vi "Hitronics.Main.vi"() -> ()   [LabVIEW 2020]
uses:
  VarsIn.ctl
  VarsOut.ctl
  State.ctl
  Agilent 2000 3000 X-Series/Agilent 2000 3000 X-Series.lvlib
panel:
  out "VarsOut":T1 {"Pk-Pk" format="%_6f"; "Delay 1-2" format="%_6f"; "Rise" format="%_6f"; "Width" format="%_6f"; "Power Value#2" format="%_6f"; "Power Value#1" format="%_6f"}
  out "error out":errorcluster
  in  "error in (no error)":errorcluster
  in  "VarsIn":T2 {"Pk-Pk" format="%_6f"; "Delay 1-2" format="%_6f"; "Rise" format="%_6f"; "Width" format="%_6f"; "Power Value#2" format="%_6f"; "Power Value#1" format="%_6f"}
  in  "Stop":bool
  in  "Test":bool=TRUE
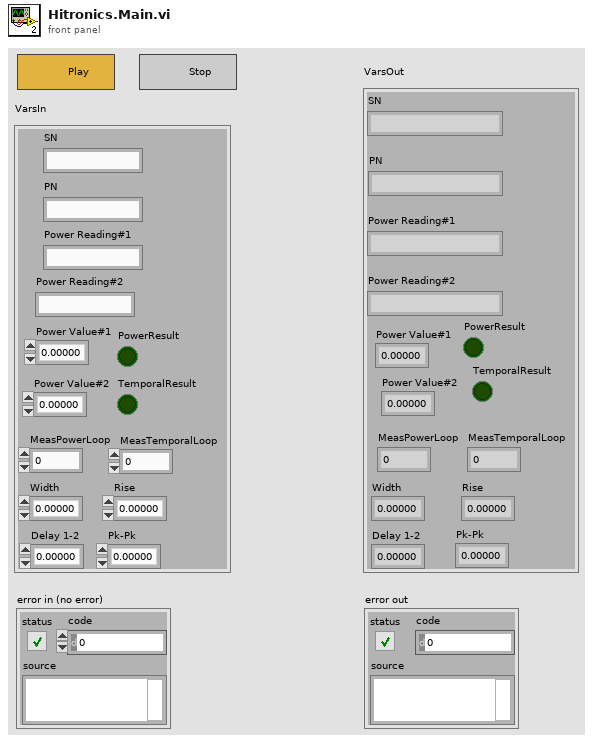
[diagram p1: front panel]
types:
  T1 = typedef "VarsOut.ctl" = cluster{"Power Reading#1":string, "Power Reading#2":string, "SN":string, "PN":string, "Power Value#1":dbl, "Power Value#2":dbl, "MeasPowerLoop":i16, "PowerResult":bool, "Width":dbl, "Rise":dbl, "Delay 1-2":dbl, "Pk-Pk":dbl, "TemporalResult":bool, "MeasTemporalLoop":i16}
  T2 = typedef "VarsIn.ctl" = cluster{"Power Reading#1":string, "Power Reading#2":string, "SN":string, "PN":string, "Power Value#1":dbl, "Power Value#2":dbl, "MeasPowerLoop":i16, "PowerResult":bool, "Width":dbl, "Rise":dbl, "Delay 1-2":dbl, "Pk-Pk":dbl, "TemporalResult":bool, "MeasTemporalLoop":i16}
  T3 = typedef "State.ctl" = enum16{"Init GUI", "ScanLabel", "MeasPower", "CheckPower", "MeasTemporal", "CheckTemporal", "Results", "SaveTestLog", "Close", "Open", "Process"}
  T4 = enum32{"invalid app kind", "Development System", "Run Time System", "Student Edition", "Embedded LabVIEW", "Evaluation", "Custom"}
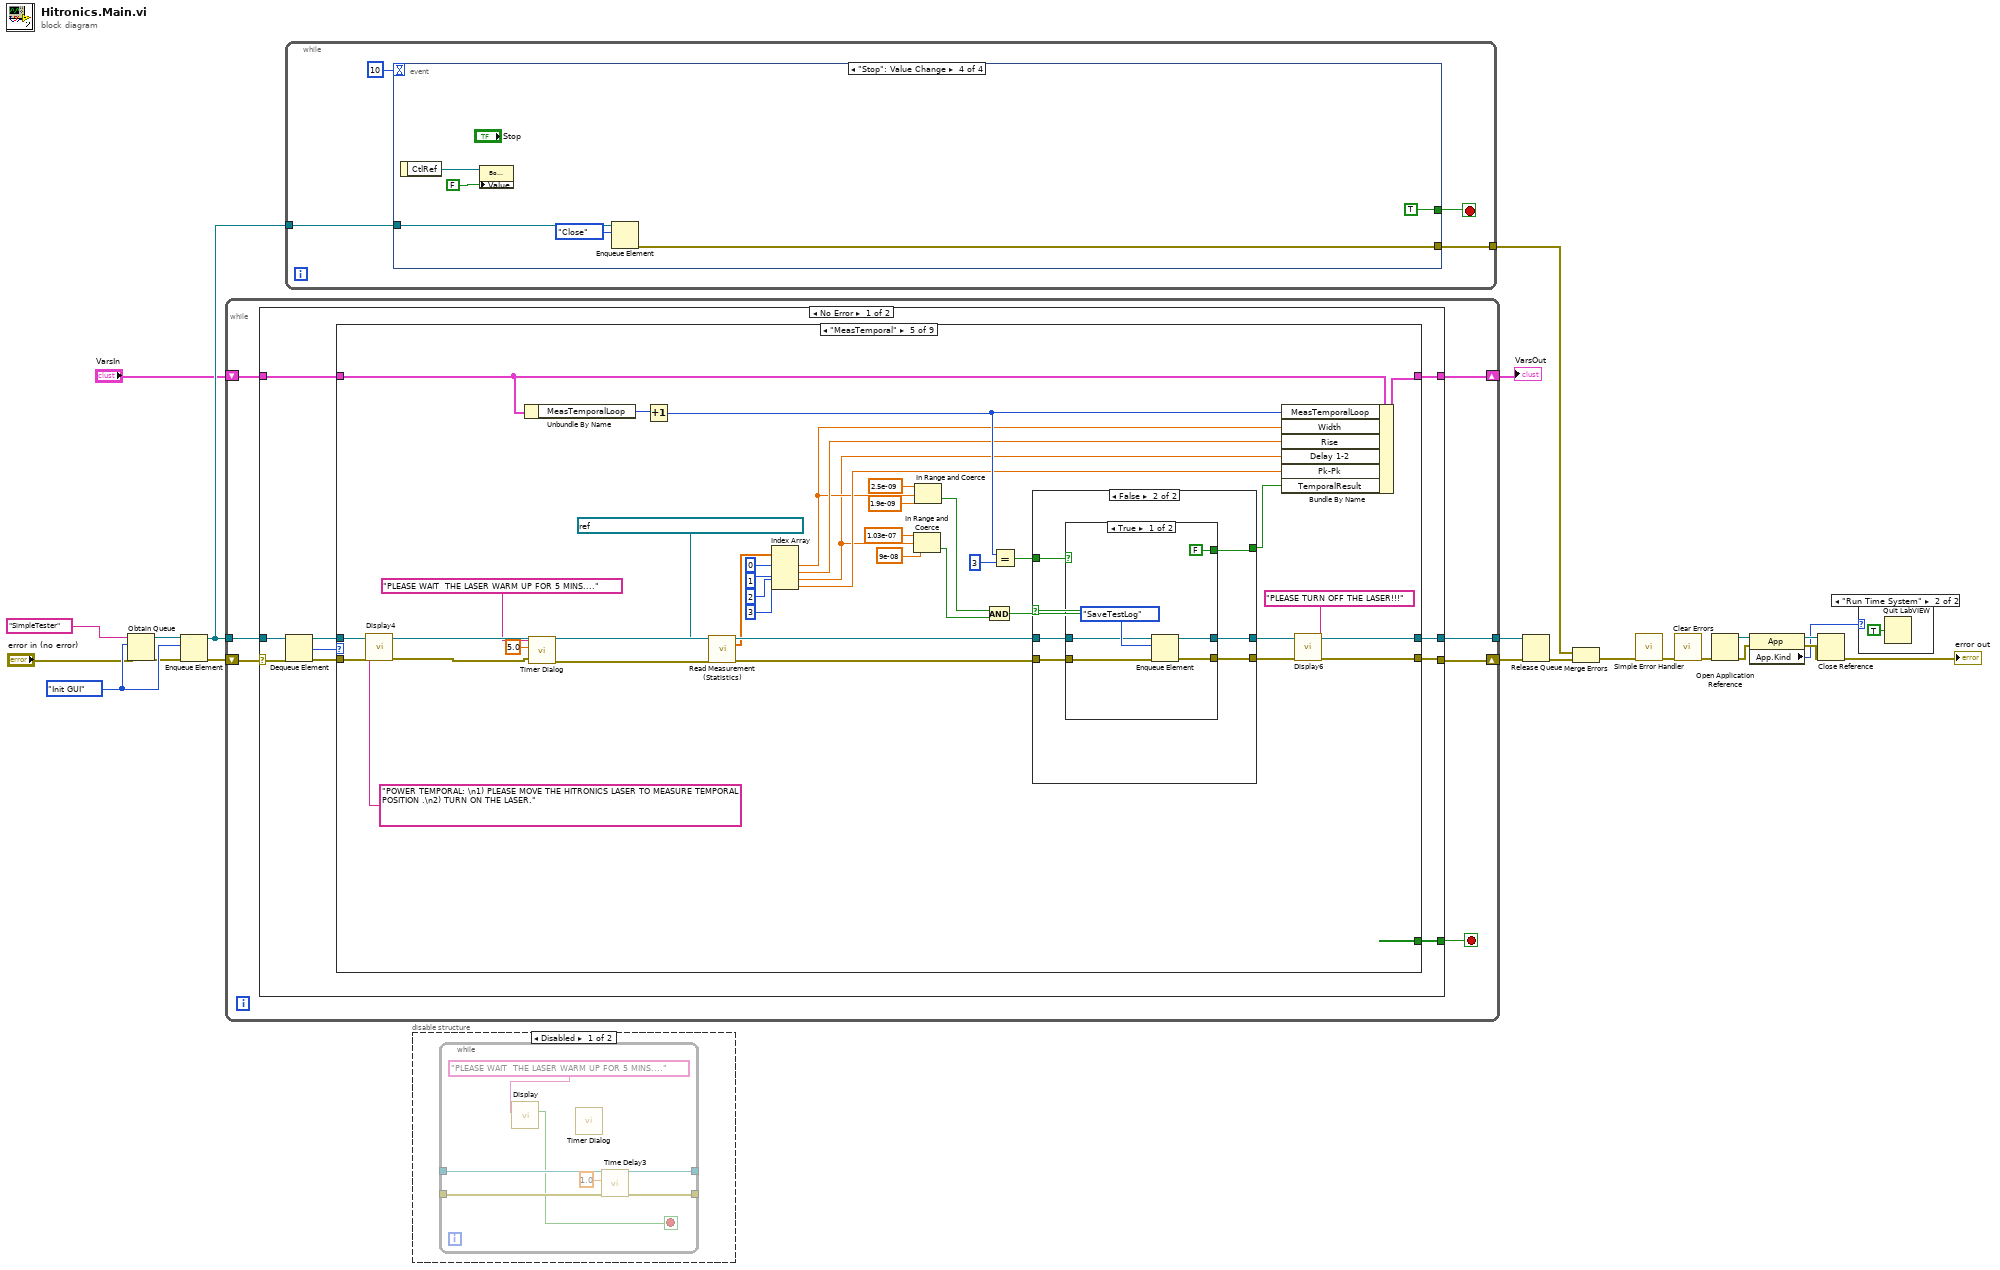
[diagram p0: block diagram]
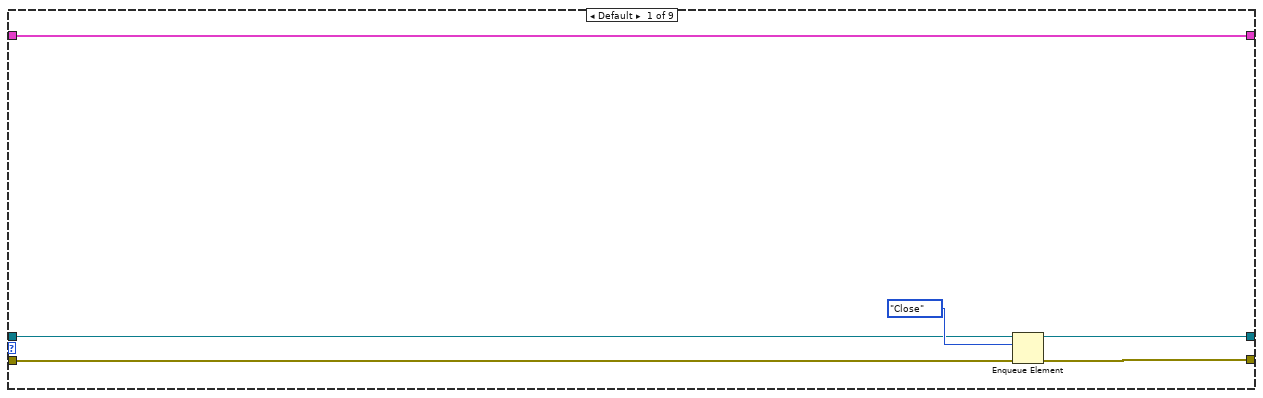
[diagram p4: hidden frame]
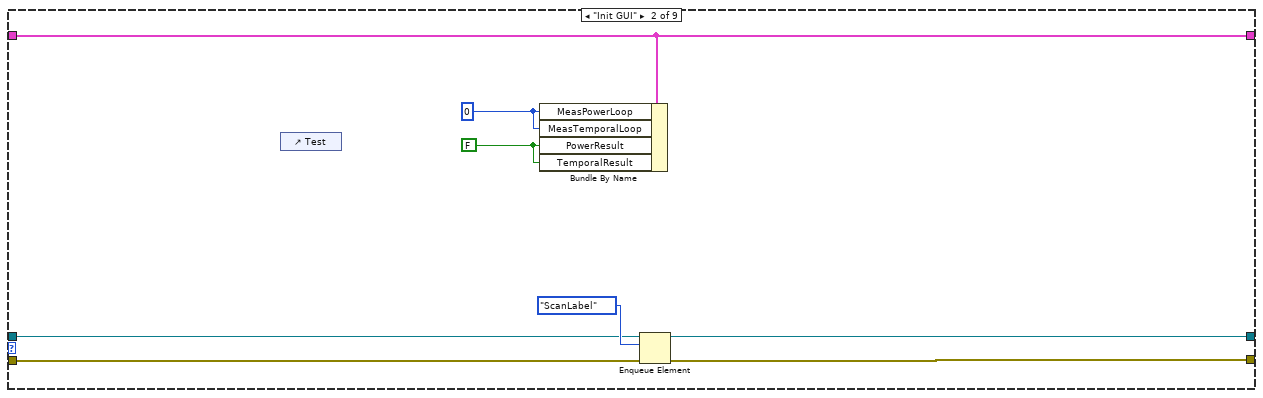
[diagram p5: hidden frame]
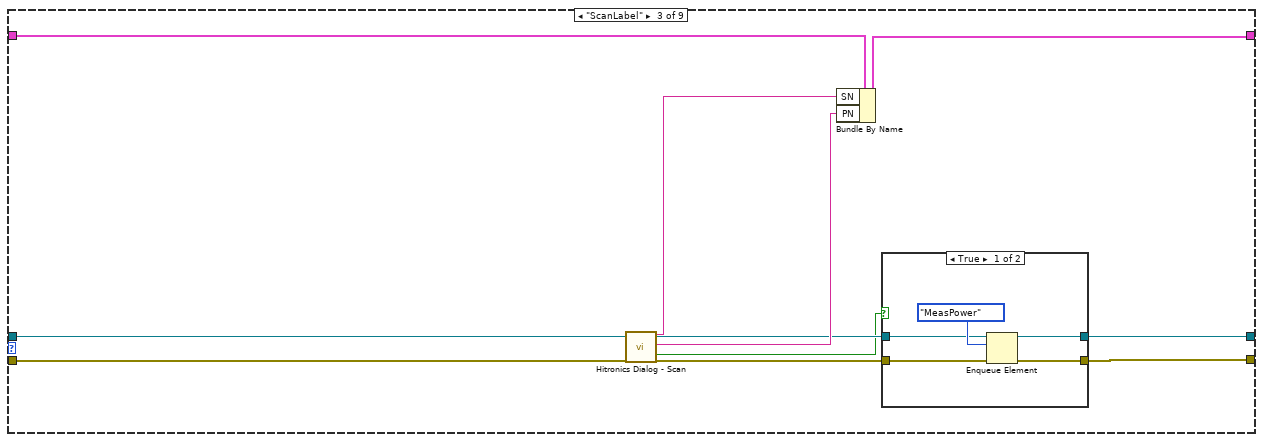
[diagram p6: hidden frame]
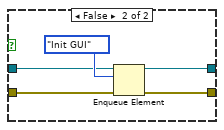
[diagram p7: hidden frame]
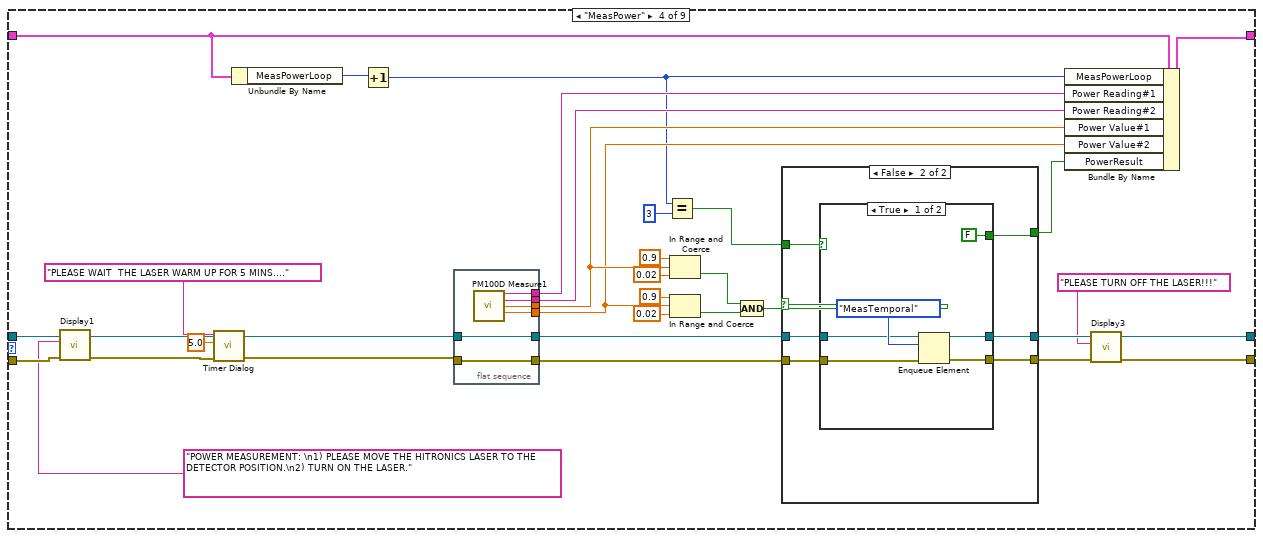
[diagram p8: hidden frame]
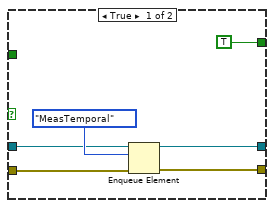
[diagram p9: hidden frame]
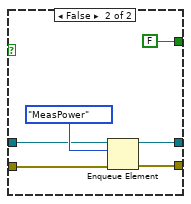
[diagram p10: hidden frame]
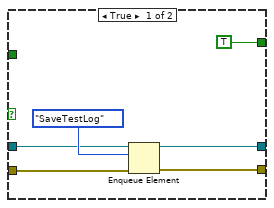
[diagram p11: hidden frame]
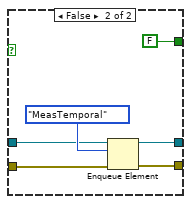
[diagram p12: hidden frame]
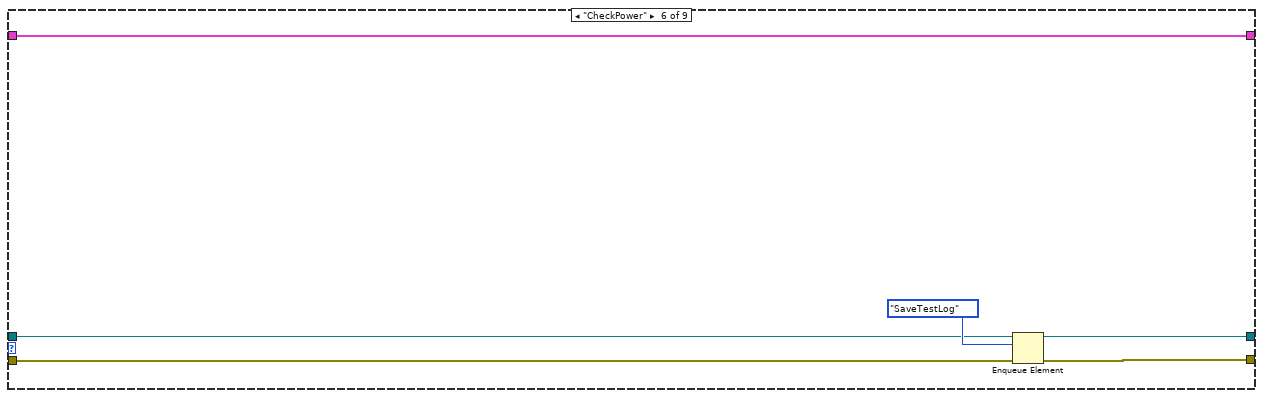
[diagram p13: hidden frame]
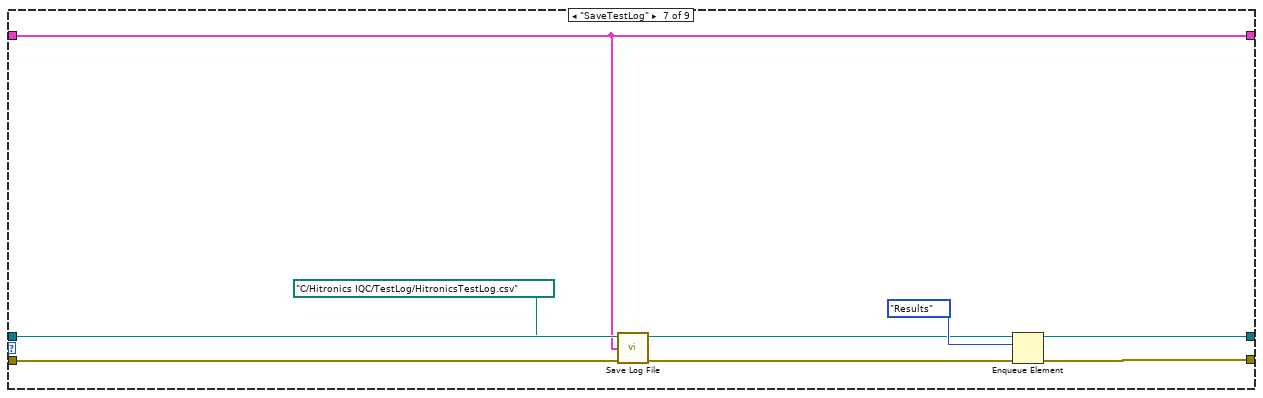
[diagram p14: hidden frame]
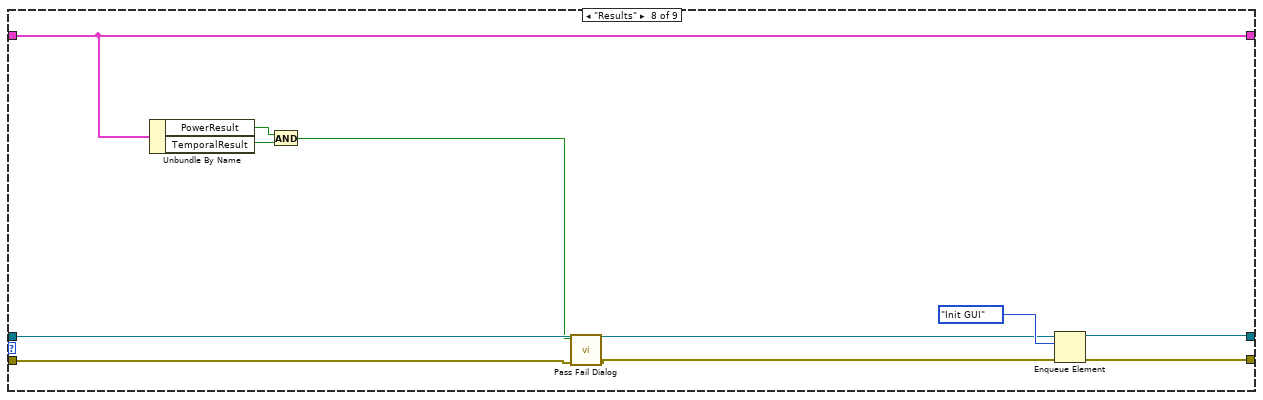
[diagram p15: hidden frame]
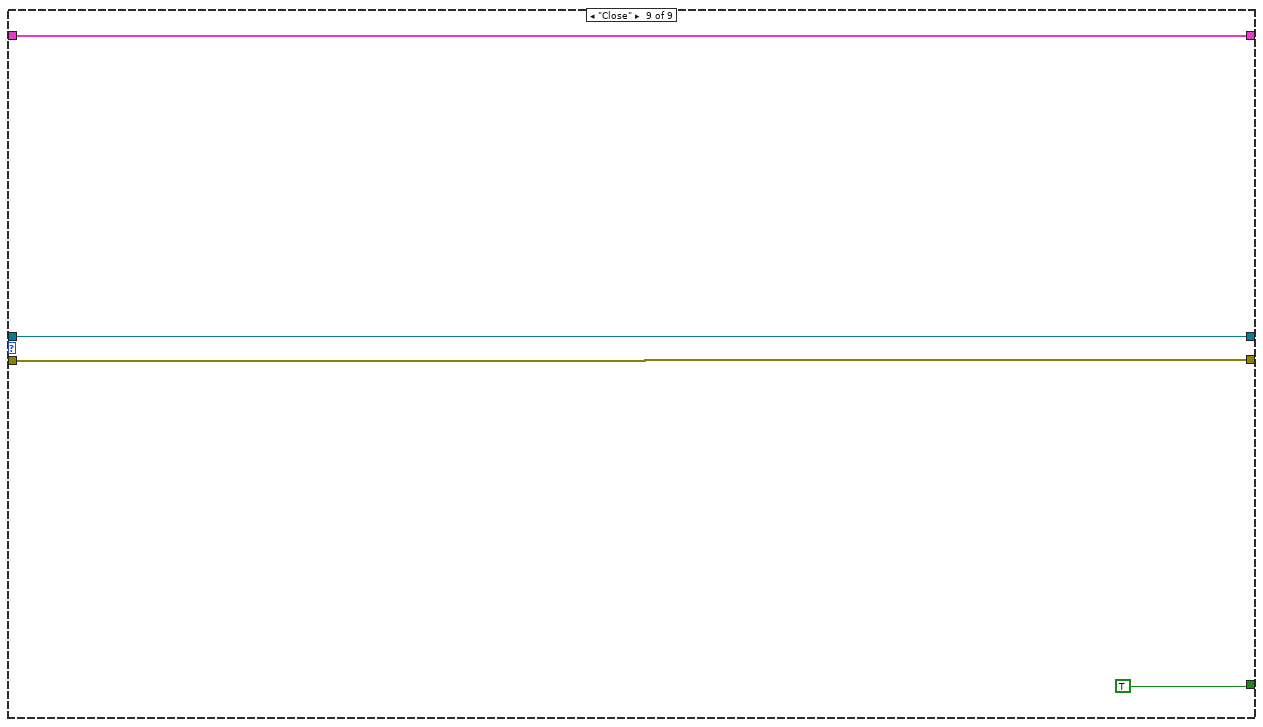
[diagram p16: hidden frame]
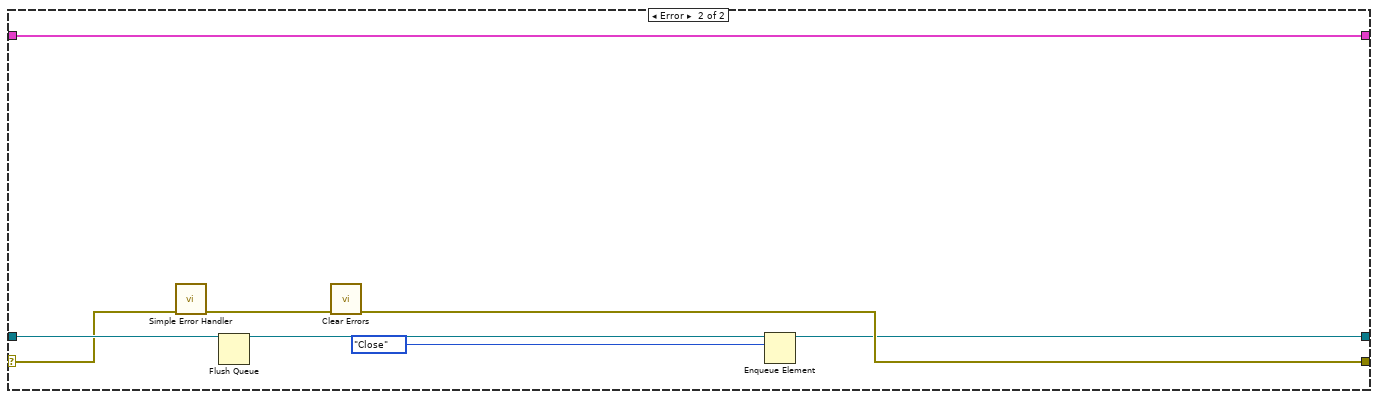
[diagram p17: hidden frame]
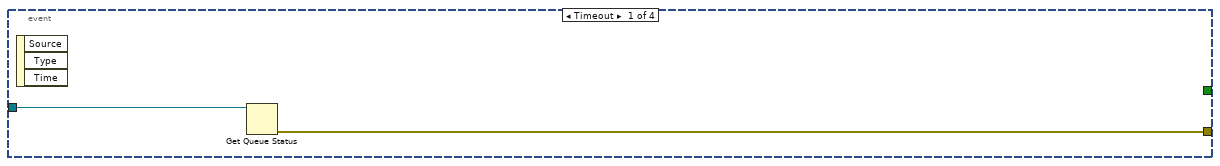
[diagram p18: hidden frame]
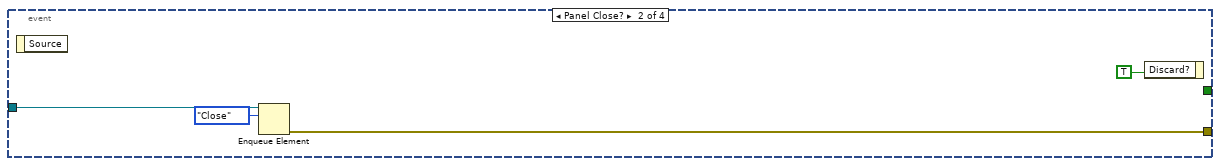
[diagram p19: hidden frame]
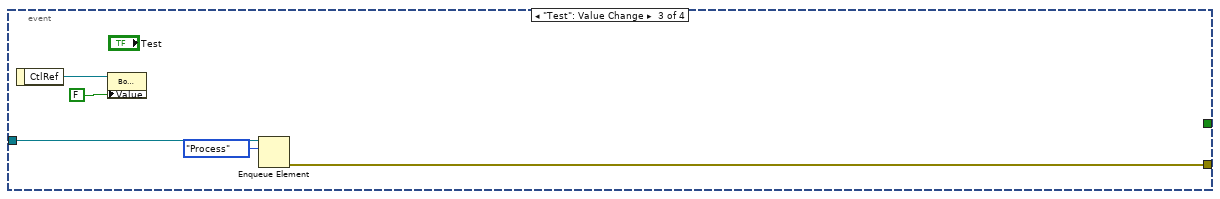
[diagram p20: hidden frame]
diagram:
  w12 = State."Init GUI"
  n1 = Obtain Queue(name (unnamed)="SimpleTester", element data type=w12, error in (no error)="error in (no error)") -> (queue out=w21:refnum<queue>, error out=w3:errorcluster)  [unwired: 2 in, 1 out]
  n2 = Enqueue Element(queue=w21, element=w12, error in (no error)=w3) -> (queue out=w19:refnum<queue>, error out=w4:errorcluster)  [unwired: 1 in, 1 out]
  n3 = while {
    tunnel: [w28] -> w20
    tunnel: w19 -> [w29]
    shift-right: [w25] -> w5
    shift-left: w4 -> [w26]
    shift-right: [w23] -> w1
    shift-left: "VarsIn" -> [w24]
    stop <- w27 stop-if-true
    n4 = case shown="No Error" w26 {
      selector: w26 -> [w32 w229]
      tunnel: w29 -> [w39 w230]
      tunnel: [w38 w224] -> w28
      tunnel: [w35 _] -> w27
      tunnel: [w30 w227] -> w25
      tunnel: [w34 w223] -> w23
      tunnel: w24 -> [w33 w223]
      frame No Error {
        n5 = Dequeue Element(queue=w39, error in (no error)=w32) -> (queue out=w37:refnum<queue>, element=w36:T3, error out=w31:errorcluster)  [unwired: 1 in, 1 out]
        n6 = case shown="\"MeasTemporal\"" w36 {
          tunnel: [w40 w49 w55 w104 w170 w197 w205 w216 w222] -> w38
          tunnel: w37 -> [w41 w50 w56 w76 w169 w198 w206 w212 w222]
          tunnel: [_ _ _ _ _ _ _ _ TRUE] -> w35
          tunnel: [w45 w48 w61 w101 w168 w196 w202 w215 w220] -> w34
          tunnel: w33 -> [w45 w48 w62 w87 w165 w196 w202 w215 w220]
          tunnel: w31 -> [w43 w52 w63 w98 w139 w195 w204 w214 w219]
          tunnel: [w42 w51 w57 w80 w140 w199 w207 w218 w219] -> w30
          frame Default {
            n7 = Enqueue Element(queue=w41, element=State."Close", error in (no error)=w43) -> (queue out=w40:refnum<queue>, error out=w42:errorcluster)  [unwired: 1 in, 1 out]
          }
          frame "Init GUI" {
            w46 = FALSE ("PowerResult")
            w47 = 0 ("MeasPowerLoop")
            n8 = control-ref of="Test"() -> ()  [unwired: 1 out]
            n9 = Bundle By Name(cluster=w48, "MeasPowerLoop"=w47, "MeasTemporalLoop"=w47, "PowerResult"=w46, "TemporalResult"=w46) -> ()  [unwired: 1 out]
            n10 = Enqueue Element(queue=w50, element=State."ScanLabel", error in (no error)=w52) -> (queue out=w49:refnum<queue>, error out=w51:errorcluster)  [unwired: 1 in, 1 out]
          }
          frame "ScanLabel" {
            n11 = call "Hitronics Dialog - Scan.vi"("error in (no error)"=w63) -> ("Serial Number"=w60:string, "Part Number"=w59:string, "Continue Exec?"=w54:bool, "error out"=w58:errorcluster)  [unwired: 14 in, 1 out]
            n12 = Bundle By Name(cluster=w62, "SN"=w60, "PN"=w59) -> (w61:T2)
            n13 = case shown="True" w54 {
              tunnel: w58 -> [w67 w72]
              tunnel: [w66 w71] -> w57
              tunnel: w56 -> [w65 w70]
              tunnel: [w64 w69] -> w55
              frame True {
                n14 = Enqueue Element(queue=w65, element=State."MeasPower", error in (no error)=w67) -> (queue out=w64:refnum<queue>, error out=w66:errorcluster)  [unwired: 1 in, 1 out]
              }
              frame False {
                n15 = Enqueue Element(queue=w70, element=State."Init GUI", error in (no error)=w72) -> (queue out=w69:refnum<queue>, error out=w71:errorcluster)  [unwired: 1 in, 1 out]
              }
            }
          }
          frame "MeasPower" {
            n16 = call "Display1"("error in (no error)"=w98, "Message"="POWER MEASUREMENT: \n1) PLEASE MOVE THE HITRONICS LASER TO THE DETECTOR POSITION.\n2) TURN ON THE LASER.") -> ("error out"=w78:errorcluster)  [unwired: 8 in, 1 out]
            n17 = call "Timer Dialog.vi"("error in (no error)"=w78, "Timeout"=5.0, "Message In"="PLEASE WAIT  THE LASER WARM UP FOR 5 MINS....") -> ("error out"=w77:errorcluster)  [unwired: 7 in, 1 out]
            n18 = Unbundle By Name(w87) -> ("MeasPowerLoop"=w86:i16)
            n19 = Increment(x=w86) -> (x+1=w85:i16)
            n20 = flat-sequence {
              tunnel: w76 -> [w134]
              tunnel: [w134] -> w103
              tunnel: w77 -> [w133]
              tunnel: [w133] -> w102
              tunnel: [w132] -> w100
              tunnel: [w131] -> w99
              tunnel: [w130] -> w96
              tunnel: [w129] -> w89
              frame #0 {
                n21 = call "PM100D Measure1.vi"() -> ("Read Power#1"=w132:string, "Read Power#2"=w131:string, "Readout value#1"=w130:dbl, "Readout value#2"=w129:dbl)  [unwired: 12 in]
              }
            }
            n22 = Equal?(x=w85, y=i16 3) -> (x = y?=w83:bool)
            n23 = In Range and Coerce(upper limit=0.9, x=w96, lower limit=0.02) -> (In Range?=w93:bool)  [unwired: 1 out]
            n24 = In Range and Coerce(upper limit=0.9, x=w89, lower limit=0.02) -> (In Range?=w88:bool)  [unwired: 1 out]
            n25 = Compound Arithmetic op=AND(w93, w88) -> (w92:bool)
            n26 = case shown="False" w92 {
              tunnel: [w109 w116] -> w79
              tunnel: [w108 w115] -> w104
              tunnel: w103 -> [w107 w114]
              tunnel: w102 -> [w106 w113]
              tunnel: w83 -> [_ w112]
              tunnel: [TRUE w111] -> w82
              frame True {
                n27 = Enqueue Element(queue=w107, element=State."MeasTemporal", error in (no error)=w106) -> (queue out=w108:refnum<queue>, error out=w109:errorcluster)  [unwired: 1 in, 1 out]
              }
              frame False {
                n28 = case shown="True" w112 {
                  tunnel: [w121 w127] -> w116
                  tunnel: [w120 w126] -> w115
                  tunnel: w114 -> [w119 w125]
                  tunnel: w113 -> [w118 w124]
                  tunnel: [FALSE FALSE] -> w111
                  frame True {
                    n29 = Enqueue Element(queue=w119, element=State."MeasTemporal", error in (no error)=w118) -> (queue out=w120:refnum<queue>, error out=w121:errorcluster)  [unwired: 1 in, 1 out]
                  }
                  frame False {
                    n30 = Enqueue Element(queue=w125, element=State."MeasPower", error in (no error)=w124) -> (queue out=w126:refnum<queue>, error out=w127:errorcluster)  [unwired: 1 in, 1 out]
                  }
                }
              }
            }
            n31 = Bundle By Name(cluster=w87, "MeasPowerLoop"=w85, "Power Reading#1"=w100, "Power Reading#2"=w99, "Power Value#1"=w96, "Power Value#2"=w89, "PowerResult"=w82) -> (w101:T2)
            n32 = call "Display3"("error in (no error)"=w79, "Message"="PLEASE TURN OFF THE LASER!!!") -> ("error out"=w80:errorcluster)  [unwired: 8 in, 1 out]
          }
          frame "MeasTemporal" {
            n33 = call "Display4"("error in (no error)"=w139, "Message"="POWER TEMPORAL: \n1) PLEASE MOVE THE HITRONICS LASER TO MEASURE TEMPORAL POSITION .\n2) TURN ON THE LASER.") -> ("error out"=w136:errorcluster)  [unwired: 8 in, 1 out]
            n34 = Unbundle By Name(w165) -> ("MeasTemporalLoop"=w164:i16)
            n35 = call "Timer Dialog.vi"("error in (no error)"=w136, "Timeout"=5.0, "Message In"="PLEASE WAIT  THE LASER WARM UP FOR 5 MINS....") -> ("error out"=w135:errorcluster)  [unwired: 7 in, 1 out]
            n36 = Increment(x=w164) -> (x+1=w163:i16)
            n37 = call "Read Measurement (Statistics).vi"("VISA resource name"=refnum<visa-resource-name> "TCPIP0::a-mx6004a-31536.local::inst0::INSTR", "error in (no error)"=w135) -> ("Mean Data"=w157:dbl[], "error out"=w159:errorcluster)  [unwired: 5 in, 7 out]
            n38 = Index Array(array=w157, index #1=0 ("index"), index #2=1 ("index"), index #3=2 ("index"), index #4=3 ("index")) -> (element #1=w149:dbl, element #2=w152:dbl, element #3=w143:dbl, element #4=w151:dbl)
            n39 = In Range and Coerce(upper limit=1.03e-07, x=w143, lower limit=9e-08 ("upper limit")) -> (In Range?=w144:bool)  [unwired: 1 out]
            n40 = In Range and Coerce(upper limit=2.5e-09, x=w149, lower limit=1.9e-09 ("upper limit")) -> (In Range?=w150:bool)  [unwired: 1 out]
            n41 = Compound Arithmetic op=AND(w150, w144) -> (w166:bool)
            n42 = Equal?(x=w163, y=i16 3) -> (x = y?=w161:bool)
            n43 = case shown="False" w166 {
              tunnel: [w175 w182] -> w141
              tunnel: [w174 w181] -> w170
              tunnel: w169 -> [w173 w180]
              tunnel: w159 -> [w172 w179]
              tunnel: w161 -> [_ w178]
              tunnel: [TRUE w177] -> w160
              frame True {
                n44 = Enqueue Element(queue=w173, element=State."SaveTestLog", error in (no error)=w172) -> (queue out=w174:refnum<queue>, error out=w175:errorcluster)  [unwired: 1 in, 1 out]
              }
              frame False {
                n45 = case shown="True" w178 {
                  tunnel: [w187 w193] -> w182
                  tunnel: [w186 w192] -> w181
                  tunnel: w180 -> [w185 w191]
                  tunnel: w179 -> [w184 w190]
                  tunnel: [FALSE FALSE] -> w177
                  frame True {
                    n46 = Enqueue Element(queue=w185, element=State."SaveTestLog", error in (no error)=w184) -> (queue out=w186:refnum<queue>, error out=w187:errorcluster)  [unwired: 1 in, 1 out]
                  }
                  frame False {
                    n47 = Enqueue Element(queue=w191, element=State."MeasTemporal", error in (no error)=w190) -> (queue out=w192:refnum<queue>, error out=w193:errorcluster)  [unwired: 1 in, 1 out]
                  }
                }
              }
            }
            n48 = Bundle By Name(cluster=w165, "MeasTemporalLoop"=w163, "Width"=w149, "Rise"=w152, "Delay 1-2"=w143, "Pk-Pk"=w151, "TemporalResult"=w160) -> (w168:T2)
            n49 = call "Display6"("error in (no error)"=w141, "Message"="PLEASE TURN OFF THE LASER!!!") -> ("error out"=w140:errorcluster)  [unwired: 8 in, 1 out]
          }
          frame "CheckPower" {
            n50 = Enqueue Element(queue=w198, element=State."SaveTestLog", error in (no error)=w195) -> (queue out=w197:refnum<queue>, error out=w199:errorcluster)  [unwired: 1 in, 1 out]
          }
          frame "SaveTestLog" {
            n51 = call "Save Log File.vi"("file path (use dialog)"=path "C:/Hitronics IQC/TestLog/HitronicsTestLog.csv", "VarsIn"=w202, "error in"=w204) -> ("error out"=w203:errorcluster)  [unwired: 12 in]
            n52 = Enqueue Element(queue=w206, element=State."Results", error in (no error)=w203) -> (queue out=w205:refnum<queue>, error out=w207:errorcluster)  [unwired: 1 in, 1 out]
          }
          frame "Results" {
            n53 = Unbundle By Name(w215) -> ("PowerResult"=w211:bool, "TemporalResult"=w210:bool)
            n54 = And(x=w211, y=w210) -> (x .and. y?=w209:bool)
            n55 = call "Pass Fail Dialog.vi"("error in (no error)"=w214, "Pass/Fail"=w209) -> ("error out"=w213:errorcluster)  [unwired: 9 in]
            n56 = Enqueue Element(queue=w212, element=State."Init GUI", error in (no error)=w213) -> (queue out=w216:refnum<queue>, error out=w218:errorcluster)  [unwired: 1 in, 1 out]
          }
          frame "Close" {
          }
        }
      }
      frame Error {
        n57 = call <vilib>:"Simple Error Handler.vi"("error in (no error)"=w229) -> ("error out"=w228:errorcluster)  [unwired: 4 in, 4 out]
        n58 = Flush Queue(queue=w230) -> (queue out=w225:refnum<queue>)  [unwired: 1 in, 2 out]
        n59 = call <vilib>:"Clear Errors.vi"("error in (no error)"=w228) -> ("error out"=w227:errorcluster)  [unwired: 5 in, 1 out]
        n60 = Enqueue Element(queue=w225, element=State."Close") -> (queue out=w224:refnum<queue>)  [unwired: 2 in, 2 out]
      }
    }
  }
  "VarsOut" <- w1
  n61 = while {
    tunnel: w19 -> [w233]
    tunnel: [w232] -> w6
    stop <- w231 stop-if-true
    n62 = event shown="[3] \"Stop\": Value Change" {
      selector: _ -> [_ _ _ _]
      dyn-events: _ -> [_ _ _ _]
      timeout: 10 -> [_ _ _ _]
      tunnel: w233 -> [w236 w239 w245 w251]
      tunnel: [w235 w238 w244 w250] -> w232
      tunnel: [_ _ _ TRUE ("Value")] -> w231
      event Timeout {
        n63 = event-data() -> ()  [unwired: 1 in, 3 out]
        n64 = Get Queue Status(queue=w236) -> (error out=w235:errorcluster)  [unwired: 2 in, 7 out]
      }
      event Panel Close? {
        n65 = event-data() -> ()  [unwired: 1 in, 1 out]
        n66 = Enqueue Element(queue=w239, element=State."Close") -> (error out=w238:errorcluster)  [unwired: 2 in, 2 out]
        n67 = event-data("Discard?"=TRUE) -> ()  [unwired: 1 in, 1 out]
      }
      event "Test": Value Change {
        n68 = event-data() -> ("CtlRef"=w242:refnum<vi>)  [unwired: 1 in]
        n69 = property class="Bool (strict)"(reference=w242, "Value"=FALSE) -> ()  [unwired: 1 in, 2 out]
        n70 = Enqueue Element(queue=w245, element=State."Process") -> (error out=w244:errorcluster)  [unwired: 2 in, 2 out]
      }
      event "Stop": Value Change {
        n71 = event-data() -> ("CtlRef"=w248:refnum<vi>)  [unwired: 1 in]
        n72 = property class="Bool (strict)"(reference=w248, "Value"=FALSE) -> ()  [unwired: 1 in, 2 out]
        n73 = Enqueue Element(queue=w251, element=State."Close") -> (error out=w250:errorcluster)  [unwired: 2 in, 2 out]
      }
    }
  }
  n74 = disable-structure shown="Disabled" {
    frame Disabled {
      n75 = while {
        tunnel: _ -> [w255]
        tunnel: [w254] -> _
        tunnel: _ -> [w257]
        tunnel: [w257] -> _
        stop <- w252 stop-if-true
        n76 = call "Display"("Message"="PLEASE WAIT  THE LASER WARM UP FOR 5 MINS....") -> ("OK"=w252:bool)  [unwired: 9 in, 1 out]
        n77 = call "Timer Dialog.vi"() -> ()  [unwired: 10 in, 2 out]
        n78 = call "Time Delay3"("error in (no error)"=w255, "Delay Time (s)"=1.0) -> ("error out"=w254:errorcluster)  [unwired: 9 in]
      }
    }
    frame Enabled {
    }
  }
  n79 = Release Queue(queue=w20, error in (no error)=w5) -> (error out=w9:errorcluster)  [unwired: 1 in, 2 out]
  n80 = Merge Errors(w6, w9) -> (w7:errorcluster)
  n81 = call <vilib>:"Simple Error Handler.vi"("error in (no error)"=w7) -> ("error out"=w8:errorcluster)  [unwired: 4 in, 4 out]
  n82 = call <vilib>:"Clear Errors.vi"("error in (no error)"=w8) -> ("error out"=w13:errorcluster)  [unwired: 5 in, 1 out]
  n83 = Open Application Reference(8:w13) -> (0:w17:errorcluster, 3:w18:refnum<vi>)  [unwired: 3 in]
  n84 = property class="App"(reference=w18, error in=w17) -> (reference out=w16:refnum<vi>, error out=w15:errorcluster, "App.Kind"=w14:T4)
  n85 = Close Reference(reference=w16, error in (no error)=w15) -> (error out=→"error out":errorcluster)
  n86 = case shown="\"Run Time System\"" w14 {
    frame "Development System", Default {
    }
    frame "Run Time System" {
      n87 = Quit LabVIEW(quit? (T)=TRUE) -> ()
    }
  }
